vi "macro_Digital_Not.vi"   [LabVIEW 2019, in "Trajectory_Library.lvlib"]
uses:
  Trajectory_Library.lvlib
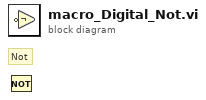
[diagram p0: block diagram]
diagram:
  # "Not"
  n1 = Not() -> ()  [unwired: 1 in, 1 out]
